vi "Main On Compile Action VI_Prepare Async_RTs RT2BC and RT2RT Words.vi"(8 "error in (no error)":errorcluster, 10 "channels":T3[](array[typedef]) {"RTs"."Mode Codes"."param item refs" format="%.0x"; "RTs"."Mode Codes"."Timestamp Channel Data Reference" format="%.0x"; "RTs"."subAddresses"."param item refs" format="%.0x"; "RTs"."subAddresses"."Timestamp Channel Data Reference" format="%.0x"; "RTs"."Status Channel Data Reference" format="%.0x"; "RTs"."Command Channels Refs" format="%.0x"; "BC"."Acyclic Frames Trigger Channels Refs" format="%.0x"; "BC"."Command Channels Refs" format="%.0x"; "BC"."messages"."Timestamp Channel Data Reference" format="%.0x"; "BC"."messages"."Status Channel Data Refs" format="%.0x"; "BC"."messages"."param item refs" format="%.0x"; "BC"."messages"."param Block Data Refs"."Data Reference" format="%.0x"}, 11 "Item Ref In":T1 format="%.0x") -> (0 "error out":errorcluster, 1 "Group":T2 {"VS Refs" format="%.0x"}, 2 "channels":T3[](array[typedef]) {"RTs"."Mode Codes"."param item refs" format="%.0x"; "RTs"."Mode Codes"."Timestamp Channel Data Reference" format="%.0x"; "RTs"."subAddresses"."param item refs" format="%.0x"; "RTs"."subAddresses"."Timestamp Channel Data Reference" format="%.0x"; "RTs"."Status Channel Data Reference" format="%.0x"; "RTs"."Command Channels Refs" format="%.0x"; "BC"."Acyclic Frames Trigger Channels Refs" format="%.0x"; "BC"."Command Channels Refs" format="%.0x"; "BC"."messages"."Timestamp Channel Data Reference" format="%.0x"; "BC"."messages"."Status Channel Data Refs" format="%.0x"; "BC"."messages"."param item refs" format="%.0x"; "BC"."messages"."param Block Data Refs"."Data Reference" format="%.0x"}, 3 "Item Ref Out":T1 format="%.0x")   [LabVIEW 2020, in "Ballard 1553 System Explorer.lvlib"]
uses:
  Ballard 1553 System Explorer.lvlib
  <vilib>/NI VeriStand/Custom Device API/Custom Device Item Ref.ctl
  Shared/Controls and Global/RT Channel.ctl
  Shared/Controls and Global/RT BC.ctl
  Shared/Controls and Global/RT Message.ctl
  Shared/Controls and Global/RT messageType.ctl
  Shared/Controls and Global/RT CWD1.ctl
  Shared/Controls and Global/RT CWD2.ctl
  <vilib>/NI VeriStand/Custom Device API/Data Reference.ctl
  <vilib>/NI VeriStand/Custom Device API/Block Data Reference.ctl
  Shared/EncodeDecode/_typedefs/parameter_config_type.ctl
  Shared/EncodeDecode/_typedefs/parameter_config_type_type.ctl
  Shared/EncodeDecode/_typedefs/parameter_config_encoding_type.ctl
  Shared/Controls and Global/RT Remote Terminal.ctl
  Shared/Controls and Global/RT Remote Terminal_rtMode.ctl
  Shared/Controls and Global/RT Remote Terminal_RT subAddress.ctl
  Shared/Controls and Global/RT Remote Terminal_RT direction.ctl
  Shared/Controls and Global/RT Remote Terminal_RT Mode Code.ctl
  <vilib>/NI VeriStand/Custom Device API/Custom Device API.lvlib
  Shared/Ballard 1553 Shared.lvlib
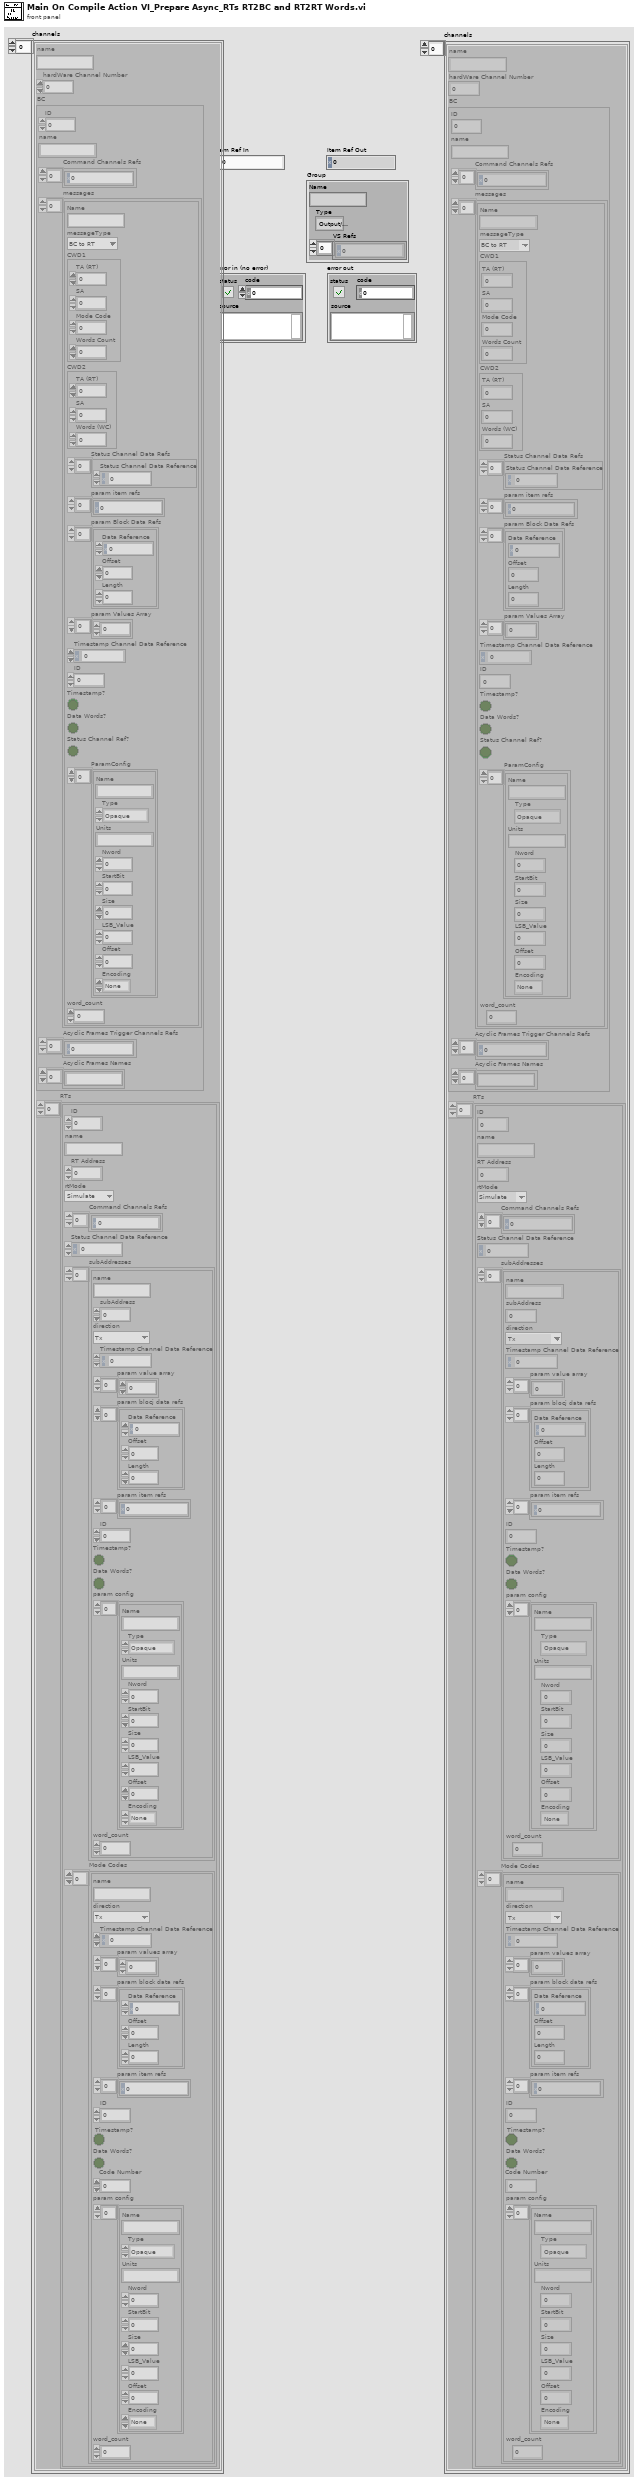
[diagram p1: front panel]
types:
  T1 = typedef "Custom Device API.lvlib/Custom Device Item Ref.ctl" = u64
  T2 = cluster{"Name":string, "Type":enum16{"Output/Write", "Input/Read", "Input/ReadWrite"}, "VS Refs":T1[]}
  T3 = typedef "Ballard 1553 Shared.lvlib/RT Channel.ctl" = cluster{"name":string, "hardWare Channel Number":u16, "BC":T4, "RTs":T14[]}
  T4 = typedef "Ballard 1553 Shared.lvlib/RT BC.ctl" = cluster{"ID":i32, "name":string, "Command Channels Refs":T1[], "messages":T5[], "Acyclic Frames Trigger Channels Refs":T1[], "Acyclic Frames Names":string[]}
  T5 = typedef "Ballard 1553 Shared.lvlib/RT Message.ctl" = cluster{"Name":string, "messageType":T6, "CWD1":T7, "CWD2":T8, "Status Channel Data Refs":T9[], "param item refs":T1[], "param Block Data Refs":T10[], "param Values Array":u16[], "Timestamp Channel Data Reference":T9, "ID":i32, "Timestamp?":bool, "Data Words?":bool, "Status Channel Ref?":bool, "ParamConfig":T11[], "word_count":u8}
  T6 = typedef "Ballard 1553 Shared.lvlib/RT messageType.ctl" = enum16{"BC to RT", "RT to BC", "RT to RT", "MC (Rx)", "MC (Tx)"}
  T7 = typedef "Ballard 1553 Shared.lvlib/RT CWD1.ctl" = cluster{"TA (RT)":i8, "SA":i8, "Mode Code":i8, "Words Count":i8}
  T8 = typedef "Ballard 1553 Shared.lvlib/RT CWD2.ctl" = cluster{"TA (RT)":i8, "SA":i8, "Words (WC)":i8}
  T9 = typedef "Custom Device API.lvlib/Data Reference.ctl" = i32
  T10 = typedef "Custom Device API.lvlib/Block Data Reference.ctl" = cluster{"Data Reference":T9, "Offset":u64, "Length":u64}
  T11 = typedef "parameter_config_type.ctl" = cluster{"Name":string, "Type":T12, "Units":string, "Nword":i32, "StartBit":i32, "Size":i32, "LSB_Value":i32, "Offset":i32, "Encoding":T13}
  T12 = typedef "parameter_config_type_type.ctl" = enum16{"Opaque", "Enum", "Float", "Integer", "Bcd", "Bool"}
  T13 = typedef "parameter_config_encoding_type.ctl" = enum16{"None", "2-complement", "Unsigned"}
  T14 = typedef "Ballard 1553 Shared.lvlib/RT Remote Terminal.ctl" = cluster{"ID":i32, "name":string, "RT Address":i32, "rtMode":T15, "Command Channels Refs":T1[], "Status Channel Data Reference":T9, "subAddresses":T16[], "Mode Codes":T18[]}
  T15 = typedef "Ballard 1553 Shared.lvlib/RT Remote Terminal_rtMode.ctl" = enum16{"Simulate", "Monitor", "Disable"}
  T16 = typedef "Ballard 1553 Shared.lvlib/RT Remote Terminal_RT subAddress.ctl" = cluster{"name":string, "subAddress":i8, "direction":T17, "Timestamp Channel Data Reference":T9, "param value array":u16[], "param blocj data refs":T10[], "param item refs":T1[], "ID":i32, "Timestamp?":bool, "Data Words?":bool, "param config":T11[], "word_count":u8}
  T17 = typedef "Ballard 1553 Shared.lvlib/RT Remote Terminal_RT direction.ctl" = enum16{"Tx", "Rx"}
  T18 = typedef "Ballard 1553 Shared.lvlib/RT Remote Terminal_RT Mode Code.ctl" = cluster{"name":string, "direction":T17, "Timestamp Channel Data Reference":T9, "param values array":u16[], "param block data refs":T10[], "param item refs":T1[], "ID":i32, "Timestamp?":bool, "Data Words?":bool, "Code Number":i32, "param config":T11[], "word_count":u8}
  T19 = enum16{"Output/Write", "Input/Read", "Input/ReadWrite"}
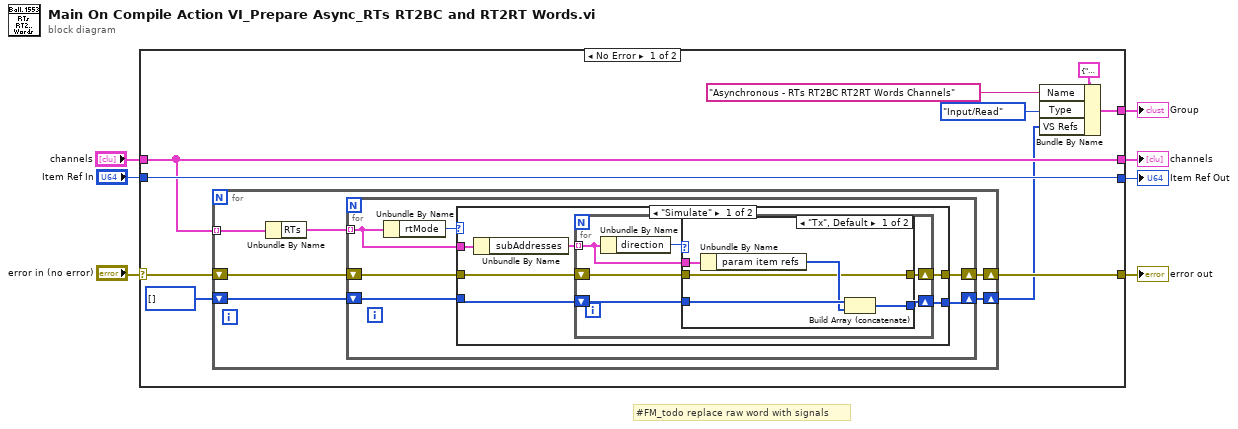
[diagram p0: block diagram]
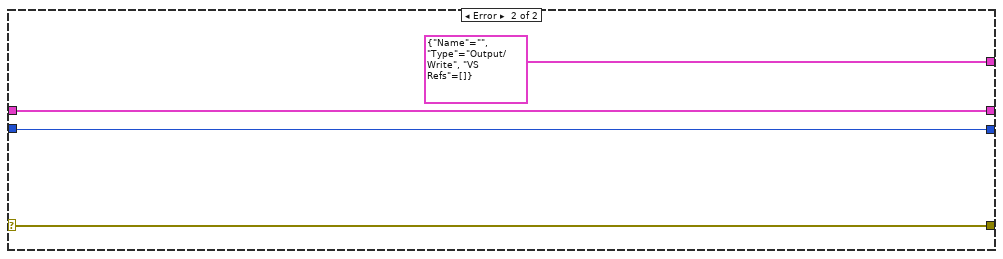
[diagram p4: hidden frame]
diagram:
  # "#FM_todo replace raw word with signals"
  n1 = case shown="No Error" "error in (no error)" {
    selector: "error in (no error)" -> [w16 w54]
    tunnel: "Item Ref In" -> [w17 w53]
    tunnel: [w14 w54] -> w5
    tunnel: "channels" -> [w15 w52]
    tunnel: [w15 w52] -> w3
    tunnel: [w17 w53] -> w2
    tunnel: [w10 T2 {"Name"="", "Type"=enum."Output/Write", "VS Refs"=[]} ("Group")] -> w1
    frame No Error {
      n2 = for {
        tunnel: w15 -> [w23] mode=indexing
        shift-right: [w18] -> w14
        shift-left: w16 -> [w20]
        shift-right: [w21] -> w11
        shift-left: T1[] [] -> [w22]
        n3 = Unbundle By Name(w23) -> ("RTs"=w19:T14[])
        n4 = for {
          shift-right: [w28] -> w21
          shift-left: w22 -> [w29]
          shift-right: [w25] -> w18
          shift-left: w20 -> [w26]
          tunnel: w19 -> [w24] mode=indexing
          n5 = Unbundle By Name(w24) -> ("rtMode"=w27:T15)
          n6 = case shown="\"Simulate\"" w27 {
            tunnel: w29 -> [w34 w49]
            tunnel: [w33 w49] -> w28
            tunnel: w26 -> [w31 w50]
            tunnel: [w30 w50] -> w25
            tunnel: w24 -> [w35 _]
            frame "Simulate" {
              n7 = Unbundle By Name(w35) -> ("subAddresses"=w32:T16[])
              n8 = for {
                tunnel: w32 -> [w36] mode=indexing
                shift-right: [w37] -> w30
                shift-left: w31 -> [w38]
                shift-right: [w40] -> w33
                shift-left: w34 -> [w41]
                n9 = Unbundle By Name(w36) -> ("direction"=w39:T17)
                n10 = case shown="\"Tx\", Default" w39 {
                  tunnel: w41 -> [w46 w47]
                  tunnel: [w45 w47] -> w40
                  tunnel: w38 -> [w42 w48]
                  tunnel: [w42 w48] -> w37
                  tunnel: w36 -> [w44 _]
                  frame "Tx", Default {
                    n11 = Unbundle By Name(w44) -> ("param item refs"=w43:T1[])
                    n12 = Build Array (concatenate)(w46, w43) -> (w45:T1[])
                  }
                  frame "Rx" {
                  }
                }
              }
            }
            frame "Monitor", Default {
            }
          }
        }
      }
      n13 = Bundle By Name(cluster=T2 {"Name"="", "Type"=enum."Output/Write", "VS Refs"=[]} ("Group"), "Name"="Asynchronous - RTs RT2BC RT2RT Words Channels", "Type"=T19."Input/Read", "VS Refs"=w11) -> (w10:T2)
    }
    frame Error {
    }
  }
  "error out" <- w5
  "Item Ref Out" <- w2
  "channels" <- w3
  "Group" <- w1
